vi "ResetTablesToTopPosition.vi"(8 "Error In":errorcluster, 11 "Table Refnum Array":refnum<vi>[](array[refnum])) -> (0 "Error Out":errorcluster)   [LabVIEW 2017, in "Client.lvlib" / "UI_API.lvlib"]
uses:
  UI_API.lvlib
  <vilib>/Utility/miscctls.llb/LVRowAndColumnUnsignedTypeDef.ctl
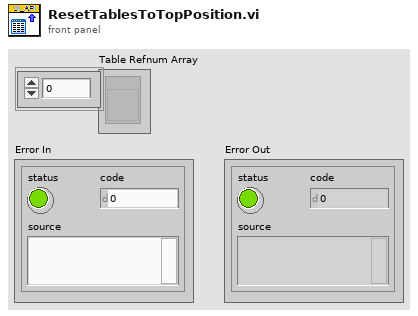
[diagram p1: front panel]
types:
  T1 = typedef "LVRowAndColumnUnsignedTypeDef.ctl" = cluster{"Row":u32, "Column":u32}
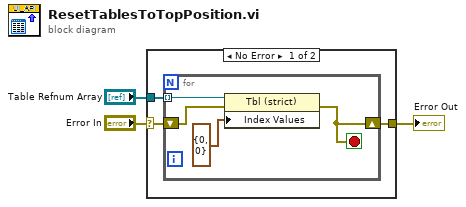
[diagram p0: block diagram]
diagram:
  n1 = case shown="No Error" "Error In" {
    selector: "Error In" -> [w5 w11]
    tunnel: "Table Refnum Array" -> [w6 _]
    tunnel: [w4 w11] -> w1
    frame No Error {
      n2 = for {
        tunnel: w6 -> [w10] mode=indexing
        shift-right: [w7] -> w4
        shift-left: w5 -> [w8]
        stop <- w7 stop-if-true
        n3 = property class="Tbl (strict)"(reference=w10, error in=w8, "Index Values"=T1 {"Row"=0, "Column"=0}) -> (error out=w7:errorcluster)  [unwired: 1 out]
      }
    }
    frame Error {
    }
  }
  "Error Out" <- w1
